vi "Test.vi"() -> ()   [LabVIEW 2020]
uses:
  SingleA/SingleA.lvclass
  SingleB/SingleB.lvclass
panel:
  in  "stop":bool
  out "value 2":string
  out "value":dbl
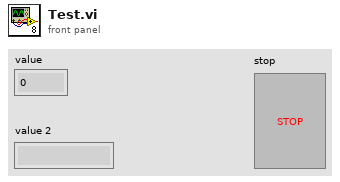
[diagram p1: front panel]
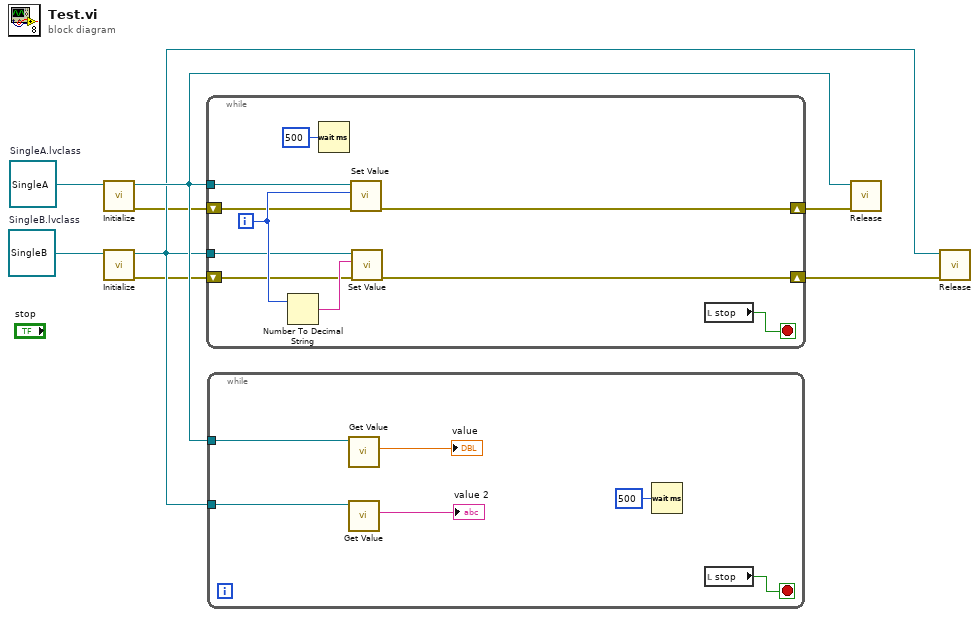
[diagram p0: block diagram]
diagram:
  w7 = refnum<class "SingleB.lvclass"> refnum  # SingleB.lvclass
  w8 = refnum<class "SingleA.lvclass"> refnum  # SingleA.lvclass
  n1 = call-dynamic "Initialize.vi"("SingleA in"=w8) -> ("error out"=w4:errorcluster, "SingleA out"=w6:refnum<class "SingleA.lvclass">)  [unwired: 9 in]
  n2 = call-dynamic "Initialize.vi"("SingleB in"=w7) -> ("error out"=w3:errorcluster, "SingleB out"=w5:refnum<class "SingleB.lvclass">)  [unwired: 9 in]
  n3 = while {
    tunnel: w6 -> [w17]
    tunnel: w5 -> [w15]
    shift-right: [w12] -> w2
    shift-left: w4 -> [w13]
    shift-right: [w10] -> w1
    shift-left: w3 -> [w11]
    i -> [w16]
    stop <- w9 stop-if-true
    n4 = Number To Decimal String(number=w16) -> (decimal integer string=w14:string)  [unwired: 1 in]
    n5 = Wait (ms)(milliseconds to wait=u32 500) -> ()  [unwired: 1 out]
    n6 = call "Set Value.vi"("error in (no error)"=w13, "value"=w16, "SingleA in"=w17) -> ("error out"=w12:errorcluster)  [unwired: 7 in, 1 out]
    n7 = call "Set Value.vi"("error in (no error)"=w11, "value"=w14, "SingleB in"=w15) -> ("error out"=w10:errorcluster)  [unwired: 7 in, 1 out]
    n8 = local read "stop"() -> (w9:bool)
  }
  n9 = while {
    tunnel: w6 -> [w23]
    tunnel: w5 -> [w21]
    stop <- w19 stop-if-true
    n10 = call "Get Value.vi"("SingleA in"=w23) -> ("value"=→"value":dbl)  [unwired: 8 in, 2 out]
    n11 = call "Get Value.vi"("SingleB in"=w21) -> ("value"=→"value 2":string)  [unwired: 8 in, 2 out]
    n12 = Wait (ms)(milliseconds to wait=u32 500) -> ()  [unwired: 1 out]
    n13 = local read "stop"() -> (w19:bool)
  }
  n14 = call-dynamic "Release.vi"("error in (no error)"=w2, "SingleA in"=w6) -> ()  [unwired: 8 in, 2 out]
  n15 = call-dynamic "Release.vi"("error in (no error)"=w1, "SingleB in"=w5) -> ()  [unwired: 8 in, 2 out]
